vi "Test List All Case Frames.vi"(8 "error in (no error)":errorcluster) -> (0 "error out":errorcluster)   [LabVIEW 2013, in "JKI State Machine API - Tests.lvlib"]
uses:
  JKI State Machine API - Tests.lvlib
  <vilib>/addons/_JKI Toolkits/Caraya/classes/Assert/Assert.lvclass
  <vilib>/addons/_JKI Toolkits/Caraya/classes/Test/Test.lvclass
  source/JKI SM/JKI SM.lvclass
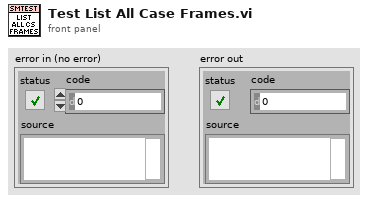
[diagram p1: front panel]
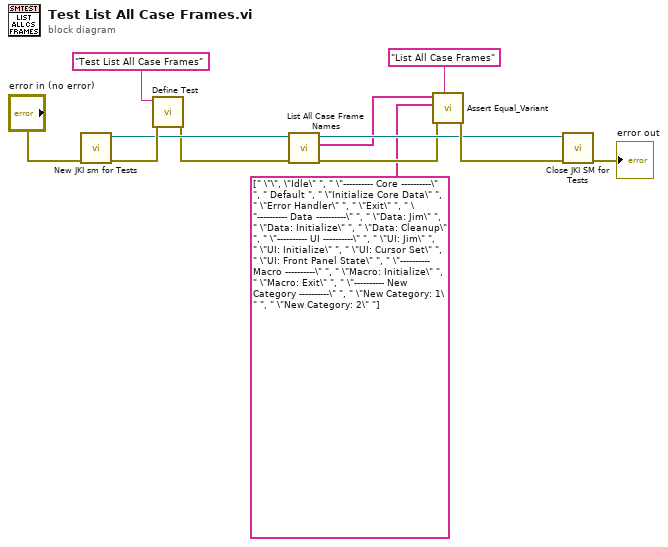
[diagram p0: block diagram]
diagram:
  n1 = call "New JKI sm for Tests.vi"("error in (no error)"="error in (no error)") -> ("error out"=w12:errorcluster, "JKI SM out"=w6:refnum<class "JKI SM.lvclass">)  [unwired: 9 in]
  n2 = call <vilib>:"Define Test.vi"("error in (no error)"=w12, "Label (VI Title)"="Test List All Case Frames") -> ("error out"=w5:errorcluster)  [unwired: 9 in]
  n3 = call "List All Case Frame Names.vi"("error in (no error)"=w5, "JKI SM in"=w6) -> ("error out"=w3:errorcluster, "All Case Structure Frame Names"=w2:string[], "JKI SM out"=w4:refnum<class "JKI SM.lvclass">)  [unwired: 7 in]
  n4 = call <vilib>:"Assert Equal_Variant.vi"("Label"="List All Case Frames", "error in (no error)"=w3, "Y"=string[] [" \"\", \"Idle\" ", " \"---------- Core ----------\" ", " Default ", " \"Initialize Core Data\" ", " \"Error Handler\" ", " \"Exit\" ", " \"---------- Data ----------\" ", " \"Data: Jim\" ", " \"Data: Initialize\" ", " \"Data: Cleanup\" ", " \"---------- UI ----------\" ", " \"UI: Jim\" ", " \"UI: Initialize\" ", " \"UI: Cursor Set\" ", " \"UI: Front Panel State\" ", " \"---------- Macro ----------\" ", " \"Macro: Initialize\" ", " \"Macro: Exit\" ", " \"---------- New Category ----------\" ", " \"New Category: 1\" ", " \"New Category: 2\" "] ("All Case Structure Frame Names"), "X"=w2) -> ("error out"=w9:errorcluster)  [unwired: 7 in]
  n5 = call "Close JKI SM for Tests.vi"("error in (no error)"=w9, "JKI SM in"=w4) -> ("error out"=→"error out":errorcluster)  [unwired: 9 in]
